vi "Schedule.Read.vi"(7 "Data to Read":variant, 8 "error in (no error)":errorcluster, 11 "Schedule <JSON> In":string) -> (0 "error out":errorcluster, 2 "Data Out":variant, 3 "Schedule <JSON> Out":string)   [LabVIEW 2019, in "ObjectSettings.lvclass"]
uses:
  ObjectSettings.lvclass
  2196355a-07f7-4609-82c2-33151c734f5a.vi
  <vilib>/JDP Science/JSONtext/Next JSON Value.vi
  <vilib>/JDP Science/JSONtext/String Subset.vi
  <vilib>/JDP Science/JSONtext/Parsing/Advance past next JSON Value (inlined COPY).vi
  <vilib>/JDP Science/JSONtext/Parsing/Advance past whitespace.vi
  <vilib>/JDP Science/JSONtext/Parsing/Advance past String.vi
  <vilib>/JDP Science/JSONtext/Parsing/Advance past Number.vi
  <vilib>/JDP Science/JSONtext/Parsing/Advance past Line Ending.vi
  <vilib>/JDP Science/JSONtext/JSON text to Variant.vi
  <vilib>/JDP Science/JSONtext/Parsing/Parse Full Path or Item Name.vi
  <vilib>/JDP Science/JSONtext/Parsing/Advance past Array.vi
  <vilib>/JDP Science/JSONtext/Parsing/Advance past Object.vi
  <vilib>/JDP Science/JSONtext/support/Error Cluster From Code.vi
  <vilib>/JDP Science/JSONtext/Offset/Find Item Locations by Path.vi
  <vilib>/JDP Science/JSONtext/LVClass Serializer/JSONtext LVClass Serializer.lvclass
  <vilib>/JDP Science/JSONtext/JSONtext.lvlib
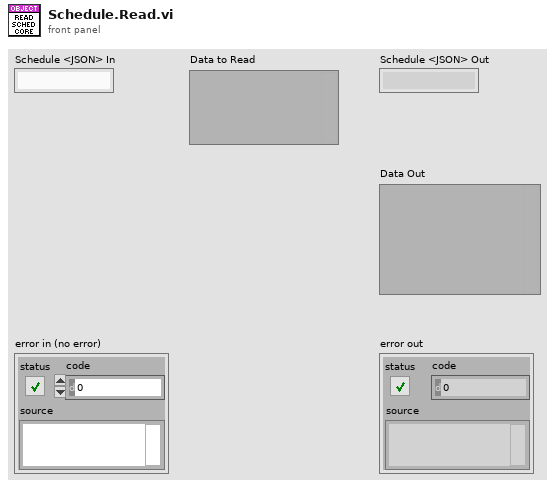
[diagram p1: front panel]
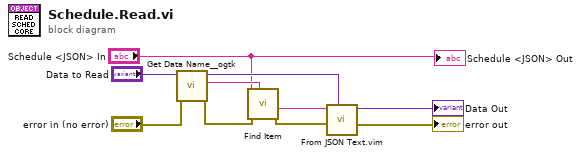
[diagram p0: block diagram]
diagram:
  n1 = call <userlib>:"Get Data Name__ogtk.vi"("error in (no error)"="error in (no error)", "Data"="Data to Read") -> ("error out"=w7:errorcluster, "Data Name"=w8:string, "Data dup"=w9:variant)  [unwired: 7 in]
  n2 = call <vilib>:"Find Item.vi"("$Path or Item Name"=w8, "error in (no error)"=w7, "JSON"="Schedule <JSON> In") -> ("error out"=w6:errorcluster, "<JSON>"=w10:string)  [unwired: 5 in, 2 out]
  n3 = call "From JSON Text.vim"("Data Type and Default Value"=w9, "error in (no error)"=w6, "JSON"=w10) -> ("error out"=→"error out":errorcluster, "Data out"=→"Data Out":variant)  [unwired: 7 in]
  "Schedule <JSON> Out" <- "Schedule <JSON> In"
